vi "run.create.request.vi"(6 "Additional Configuration":T1, 8 "error in (no error)":errorcluster, 9 "Timing":cluster{"Start":timestamp, "End":timestamp} {"End" format="%<%x %.3X>T"; "Start" format="%<%x %.3X>T"}, 10 "Titles":cluster{"Name":string, "Description":string}, 11 "Nominal Client in":refnum<class "Nominal Client.lvclass">) -> (0 "error out":errorcluster, 2 "Request Body":string, 3 "Nominal Client out":refnum<class "Nominal Client.lvclass">)   [LabVIEW 2020, in "Nominal Client.lvclass"]
uses:
  Nominal Client.lvclass
  Nominal Client.lvclass/Nominal Client.ctl
  nominal types/workspace/workspace.lvclass/workspace.ctl
  984f11ad-4b88-4f46-a0da-23de5fac9e3d.vi
  0bd34b97-91d1-4161-9f6d-cadc33e40760.vi
  2be38be4-a54f-44d4-b7cf-5ac4b5fc8952.vi
  bc98cd5f-ae14-4807-8600-5baebe045155.vi
  b56b23ec-042d-4749-be22-73137a14bf37.vi
  workspace.get.vi
  <vilib>/JDP Science/JSONtext/Merge into Object.vi
  workspace.add_to_payload.vi/88650e10-de3e-481c-85db-71cb0fdf4485.vi
  nominal types/workspace/rid.get.vi
  <vilib>/LabVIEW Open Source Project/Epoch Date & Time/epoch.UNIX/Epoch.UNIX.lvclass
  C:/Program Files/National Instruments/LabVIEW 2020/vi.lib/LabVIEW Open Source Project/Epoch Date & Time/epoch/Epoch.lvclass
  <vilib>/LabVIEW Open Source Project/Epoch Date & Time/Get Epoch Time.vi
  <vilib>/JDP Science/JSONtext/Variant to JSON Text.vi
  <vilib>/JDP Science/JSONtext/Array of Variants to JSON Object.vi
  <vilib>/JDP Science/JSONtext/Set Item.vi
  <vilib>/JDP Science/JSONtext/Get all Object Items.vi
  <vilib>/JDP Science/JSONtext/Set Multiple Object Items.vi
  <vilib>/JDP Science/JSONtext/LVClass Serializer/JSONtext LVClass Serializer.lvclass
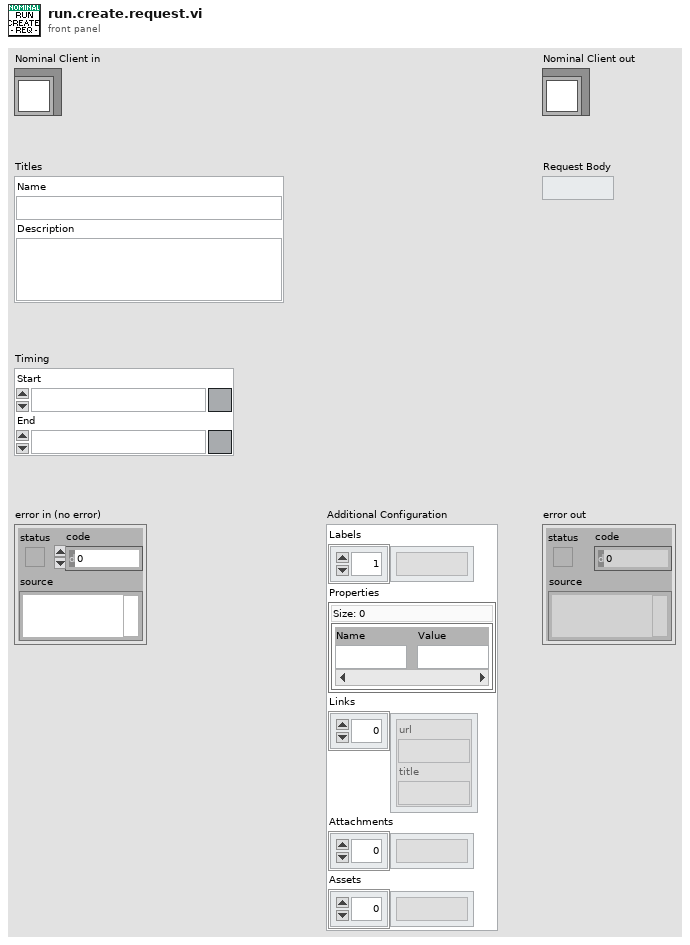
[diagram p1: front panel]
types:
  T1 = cluster{"Labels":string[], "Properties":map{string, string}, "Links":cluster{"url":string, "title":string}[], "Attachments":string[], "Assets":string[]}
  T2 = cluster{"title":string, "description":string, "startTime":cluster{"secondsSinceEpoch":i32, "offsetNanoseconds":i32}, "properties":string, "labels":string[], "links":cluster{"url":string, "title":string}[], "attachments":string[], "assets":string[]}
  T3 = cluster{"title":string, "description":string, "startTime":cluster{"secondsSinceEpoch":i32, "offsetNanoseconds":i32}, "properties":string, "labels":string[], "links":cluster{"url":string, "title":string}[], "attachments":string[], "assets":string[], "endTime":cluster{"secondsSinceEpoch":i32, "offsetNanoseconds":i32}}
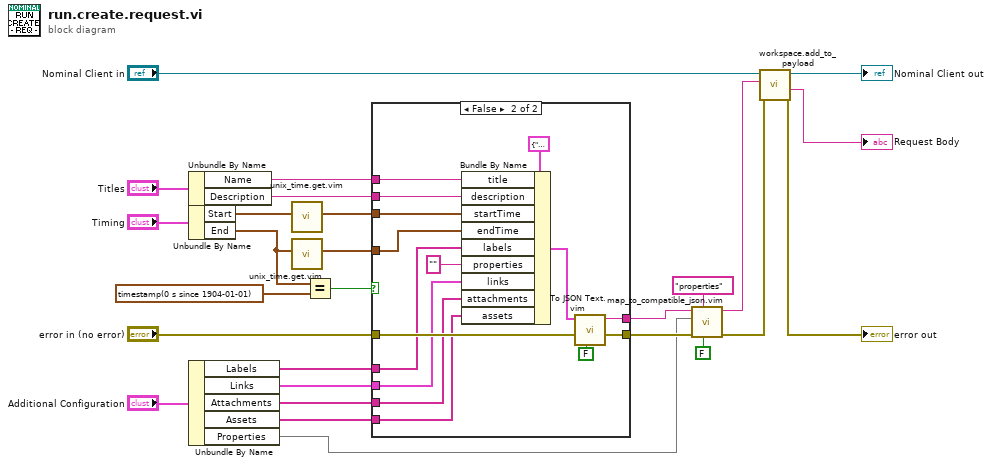
[diagram p0: block diagram]
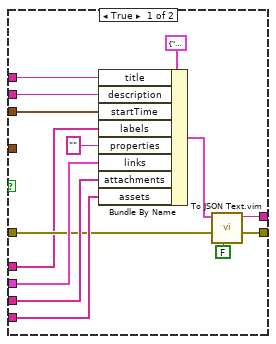
[diagram p2: hidden frame]
diagram:
  n1 = Unbundle By Name("Titles") -> ("Name"=w25:string, "Description"=w24:string)
  n2 = Unbundle By Name("Timing") -> ("Start"=w23:timestamp, "End"=w2:timestamp)
  n3 = Unbundle By Name("Additional Configuration") -> ("Labels"=w13:string[], "Links"=w21:cluster{"url":string, "title":string}[], "Attachments"=w20:string[], "Assets"=w19:string[], "Properties"=w12:map{string, string})
  n4 = call "unix_time.get.vim"("Time Stamp (empty: now) [single or array]"=w23) -> ("UNIX Timestamp"=w22:cluster{"Seconds":i64, "Nanoseconds":i64})  [unwired: 10 in]
  n5 = call "unix_time.get.vim"("Time Stamp (empty: now) [single or array]"=w2) -> ("UNIX Timestamp"=w16:cluster{"Seconds":i64, "Nanoseconds":i64})  [unwired: 10 in]
  n6 = Equal?(x=w2, y=timestamp(0 s since 1904-01-01) ("End")) -> (x = y?=w14:bool)
  n7 = case shown="False" w14 {
    tunnel: [w41 w55] -> w26
    tunnel: w25 -> [w39 w53]
    tunnel: w24 -> [w38 w52]
    tunnel: w22 -> [w37 w51]
    tunnel: w21 -> [w35 w49]
    tunnel: w20 -> [w34 w48]
    tunnel: w19 -> [w33 w47]
    tunnel: [w31 w45] -> w18
    tunnel: "error in (no error)" -> [w30 w56]
    tunnel: w13 -> [w28 w43]
    tunnel: w16 -> [_ w42]
    frame True {
      n8 = Bundle By Name(cluster=T2 {"title"="", "description"="", "startTime"={"secondsSinceEpoch"=0, "offsetNanoseconds"=0}, "properties"="", "labels"=[], "links"=[], "attachments"=[], "assets"=[]}, "title"=w39, "description"=w38, "startTime"=w37, "labels"=w28, "properties"="", "links"=w35, "attachments"=w34, "assets"=w33) -> (w32:T2)
      n9 = call "To JSON Text.vim"("Pretty Print?"=FALSE, "error in (no error)"=w30, "Anything"=w32) -> ("error out"=w31:errorcluster, "<JSON>"=w41:string)  [unwired: 7 in]
    }
    frame False {
      n10 = Bundle By Name(cluster=T3 {"title"="", "description"="", "startTime"={"secondsSinceEpoch"=0, "offsetNanoseconds"=0}, "properties"="", "labels"=[], "links"=[], "attachments"=[], "assets"=[], "endTime"={"secondsSinceEpoch"=0, "offsetNanoseconds"=0}}, "title"=w53, "description"=w52, "startTime"=w51, "endTime"=w42, "labels"=w43, "properties"="", "links"=w49, "attachments"=w48, "assets"=w47) -> (w46:T3)
      n11 = call "To JSON Text.vim"("Pretty Print?"=FALSE, "error in (no error)"=w56, "Anything"=w46) -> ("error out"=w45:errorcluster, "<JSON>"=w55:string)  [unwired: 7 in]
    }
  }
  n12 = call "map_to_compatible_json.vim"("Pretty Print?"=FALSE, "JSON Path"="properties" ("Data Name"), "error in"=w18, "Map"=w12, "JSON in"=w26) -> ("error out"=w10:errorcluster, "JSON out"=w11:string)  [unwired: 5 in]
  n13 = call "workspace.add_to_payload.vi"("error in"=w10, "JSON payload in"=w11, "Nominal Client in"="Nominal Client in") -> ("error out"=→"error out":errorcluster, "JSON payload out"=→"Request Body":string, "Nominal Client out"=→"Nominal Client out":refnum<class "Nominal Client.lvclass">)  [unwired: 6 in]
